vi "iRobot Read Charging Sources Available.vi"(11 "stream in":u8[](array[numeric])) -> (1 "Charging Sources Available":T1, 3 "stream out":u8[](array[numeric]))   [LabVIEW 2010]
doc: "Read available charging sources from a UART stream."
uses:
  Sensor Controls/iRobot Charging Sources Available.ctl
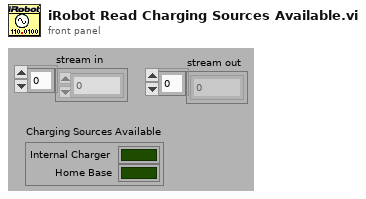
[diagram p1: front panel]
types:
  T1 = typedef "iRobot Charging Sources Available.ctl" = cluster{"Internal Charger":bool, "Home Base":bool}
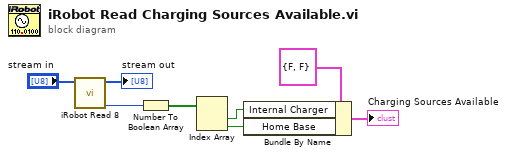
[diagram p0: block diagram]
diagram:
  n1 = call "iRobot Read 8.vi"("stream in"="stream in") -> ("value"=w4:u8, "stream out"=→"stream out":u8[])  [unwired: 9 out]
  n2 = Number To Boolean Array(number=w4) -> (Boolean array=w8:bool[])
  n3 = Index Array(array=w8) -> (element #1=w7:bool, element #2=w1:bool)  [unwired: 2 in]
  n4 = Bundle By Name(cluster=T1 {"Internal Charger"=FALSE, "Home Base"=FALSE} ("Charging Sources Available"), "Internal Charger"=w7, "Home Base"=w1) -> (→"Charging Sources Available":T1)
